vi "AssertConnectorPanesMatchExpected.vi"(8 "error in (no error)":errorcluster, 10 "custom device xml path":path, 11 "TestCase in":refnum<class "TestCase.lvclass">) -> (0 "error out":errorcluster, 3 "TestCase out":refnum<class "TestCase.lvclass">)   [LabVIEW 2027, in "VeriStandTestUtilities.lvlib"]
uses:
  VeriStandTestUtilities.lvlib
  <vilib>/addons/_JKI Toolkits/VI Tester/TestCase.llb/TestCase.lvclass
  <userlib>/_OpenG.lib/file/file.llb/Append Path to Root if Relative - Scalar__ogtk.vi
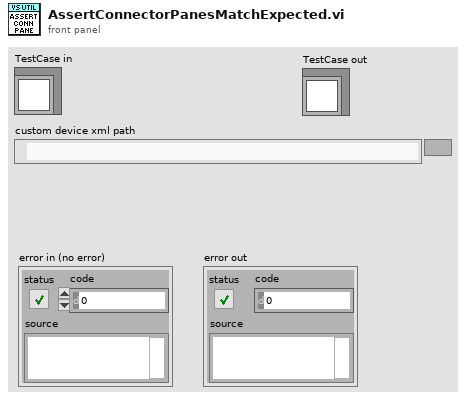
[diagram p1: front panel]
types:
  T1 = cluster{"VI Path":string, "Template File":path, "Terminal subset ok?":bool}[]
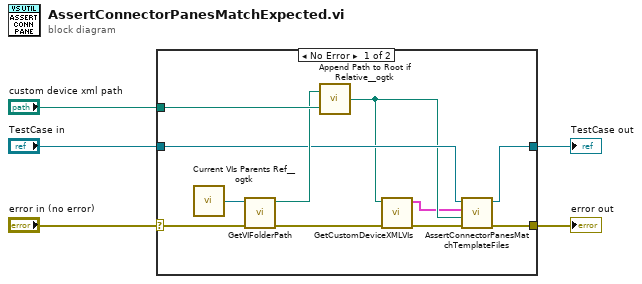
[diagram p0: block diagram]
diagram:
  n1 = case shown="No Error" "error in (no error)" {
    selector: "error in (no error)" -> [w12 w18]
    tunnel: [w15 w18] -> w5
    tunnel: "custom device xml path" -> [w16 _]
    tunnel: "TestCase in" -> [w10 w17]
    tunnel: [w14 w17] -> w1
    frame No Error {
      n2 = call <userlib>:"Current VIs Parents Ref__ogtk.vi"() -> ("Calling VI's Reference"=w13:refnum<vi>)  [unwired: 2 in]
      n3 = call "GetVIFolderPath.vi"("error in (no error)"=w12, "VI Reference in"=w13) -> ("error out"=w9:errorcluster, "VI Folder Path out"=w11:path)  [unwired: 8 in]
      n4 = call-poly <userlib>:"Append Path to Root if Relative__ogtk.vi"("Absolute or Relative Path"=w16, "Root Path"=w11) -> ("Absolute or Appended Path"=w7:path)
      n5 = call "GetCustomDeviceXMLVIs.vi"("error in (no error)"=w9, "absolute custom device xml file"=w7) -> ("error out"=w8:errorcluster, "custom device VIs"=w6:T1)  [unwired: 8 in]
      n6 = call "AssertConnectorPanesMatchTemplateFiles.vi"("error in (no error)"=w8, "absolute custom device xml file"=w7, "Array"=w6, "TestCase in"=w10) -> ("error out"=w15:errorcluster, "TestCase out"=w14:refnum<class "TestCase.lvclass">)  [unwired: 6 in]
    }
    frame Error {
    }
  }
  "error out" <- w5
  "TestCase out" <- w1
